vi "MSEditor_Script_UndoFGV.vi"(1 "Script in":string, 3 "error in (no error)":errorcluster, 4 "Function":enum16{"Write", "Read"}(ring)) -> (8 "Script out":string, 10 "error out":errorcluster)   [LabVIEW 2018]
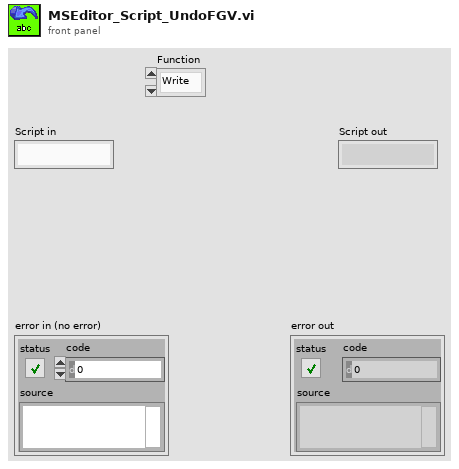
[diagram p1: front panel]
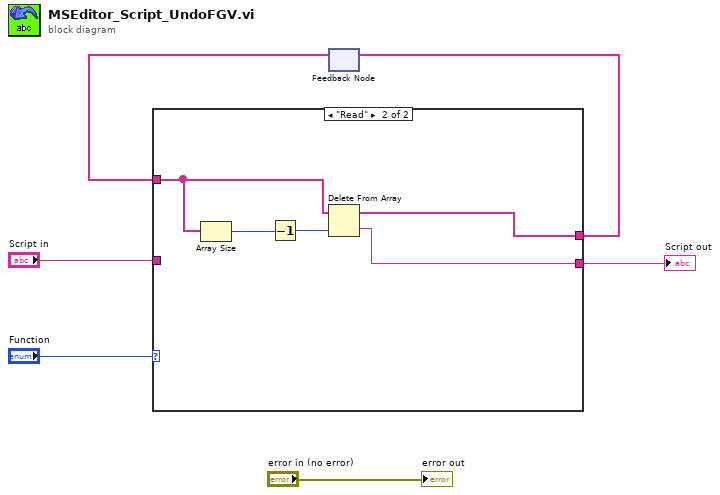
[diagram p0: block diagram]
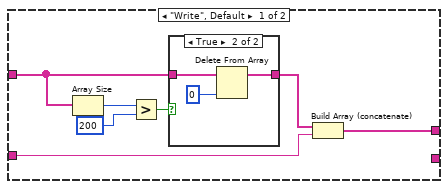
[diagram p2: hidden frame]
diagram:
  n1 = feedback #1() -> (w2:string[])  [unwired: 1 in]
  n2 = case shown="\"Read\"" "Function" {
    tunnel: "Script in" -> [w13 _]
    tunnel: [w12 w19] -> w3
    tunnel: w2 -> [w8 w22]
    tunnel: [_ w18] -> w1
    frame "Write", Default {
      n3 = Array Size(array=w8) -> (size(s)=w11:i32)
      n4 = Greater?(x=w11, y=200) -> (0:w9:bool)
      n5 = case shown="True" w9 {
        tunnel: w8 -> [w14 w17]
        tunnel: [w14 w15] -> w7
        frame False {
        }
        frame True {
          n6 = Delete From Array(array=w17, index=0) -> (array with subset deleted=w15:string[])  [unwired: 1 in, 1 out]
        }
      }
      n7 = Build Array (concatenate)(w7, w13) -> (w12:string[])
    }
    frame "Read" {
      n8 = Array Size(array=w22) -> (size(s)=w21:i32)
      n9 = Decrement(x=w21) -> (x-1=w20:i32)
      n10 = Delete From Array(array=w22, index=w20) -> (deleted portion=w18:string, array with subset deleted=w19:string[])  [unwired: 1 in]
    }
  }
  "Script out" <- w1
  n11 = feedback-in #1(w3) -> ()
  "error out" <- "error in (no error)"
